vi "CHROMA Set Voltage.vi"(7 "Phase":T1, 8 "Error In":errorcluster, 10 "Voltage Setpoint":dbl, 11 "CHROMA VISA In":refnum<visa-resource-name>) -> (0 "Error Out":errorcluster, 3 "CHROMA VISA Out":refnum<visa-resource-name>)   [LabVIEW 2016]
uses:
  Type Definition/CHROMA Phase.ctl
  Type Definition/CHROMA Build CMD Type.ctl
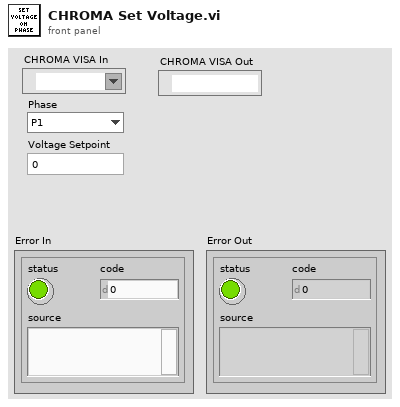
[diagram p1: front panel]
types:
  T1 = typedef "CHROMA Phase.ctl" = enum16{"P1", "P2", "P3"}
  T2 = typedef "CHROMA Build CMD Type.ctl" = enum16{"Value DBL", "Value I32", "String"}
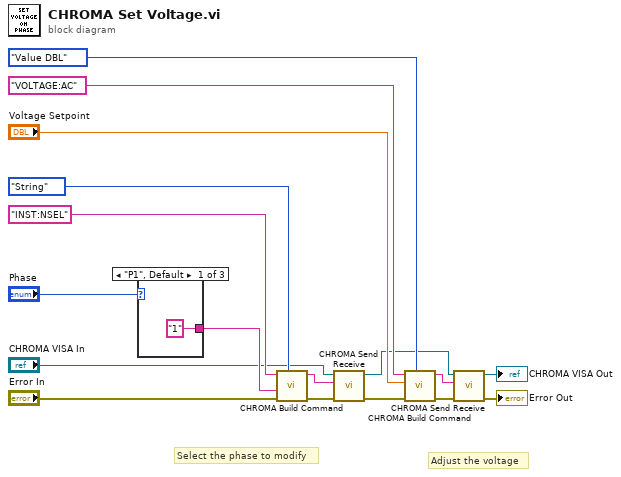
[diagram p0: block diagram]
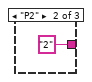
[diagram p2: hidden frame]
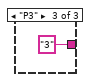
[diagram p3: hidden frame]
diagram:
  # "Adjust the voltage"
  # "Select the phase to modify"
  n1 = case shown="\"P1\", Default" "Phase" {
    tunnel: ["1" "2" "3"] -> w12
    frame "P1", Default {
    }
    frame "P2" {
    }
    frame "P3" {
    }
  }
  n2 = call "CHROMA Build Command.vi"("Build Type"=CHROMA_Build_CMD_Type."String", "Error In"="Error In", "String"=w12, "Partial Command"="INST:NSEL" ("string to write")) -> ("Error Out"=w14:errorcluster, "Chroma Command"=w15:string)  [unwired: 6 in]
  n3 = call "CHROMA Send Receive.vi"("error in (no error)"=w14, "Send Command"=w15, "CHROMA VISA In"="CHROMA VISA In") -> ("error out"=w16:errorcluster, "CHROMA VISA Out"=w7:refnum<visa-resource-name>)  [unwired: 6 in, 1 out]
  n4 = call "CHROMA Build Command.vi"("Build Type"=CHROMA_Build_CMD_Type."Value DBL", "Error In"=w16, "Value"="Voltage Setpoint", "Partial Command"="VOLTAGE:AC" ("string to write")) -> ("Error Out"=w5:errorcluster, "Chroma Command"=w6:string)  [unwired: 6 in]
  n5 = call "CHROMA Send Receive.vi"("error in (no error)"=w5, "Send Command"=w6, "CHROMA VISA In"=w7) -> ("error out"=→"Error Out":errorcluster, "CHROMA VISA Out"=→"CHROMA VISA Out":refnum<visa-resource-name>)  [unwired: 6 in, 1 out]
